vi "Get ASCII string.vi"(8 "error in (no error)":errorcluster, 11 "VISA resource name":refnum<visa-resource-name>) -> (0 "error out":errorcluster, 2 "String":string, 3 "VISA resource name out":refnum<visa-resource-name>)   [LabVIEW 2012, in "Datron D4xxx.lvlib"]
doc: "This VI returns stored ASCII string (X8 command)."
uses:
  Datron D4xxx.lvlib
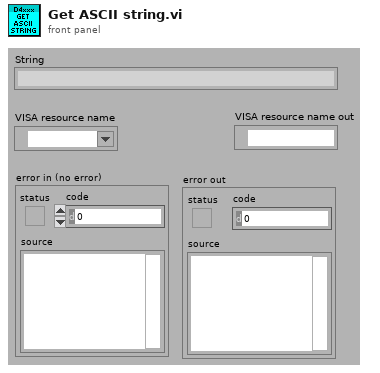
[diagram p1: front panel]
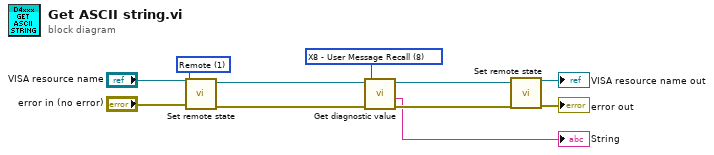
[diagram p0: block diagram]
diagram:
  w6 = u16 8 items=["X0 - Zero Cal Store", "X1 - Gain Cal Store", "X2 - STD Cal Gain Factor", "X3 - Zero Offset", "X4 - Gain Offset", "X5 - Linearity", "X6 - Reference Divider Setting", "X7 - Spot Freq. Corrections", "X8 - User Message Recall", "X9 - Recall Cal Store Selection"] ("X command (X8)")
  w7 = u16 1 items=["Local", "Remote", "Default"] ("Remote state")
  n1 = call "Set remote state.vi"("error in"="error in (no error)", "Remote state"=w7, "VISA resource name"="VISA resource name") -> ("error out"=w4:errorcluster, "VISA resource name out"=w5:refnum<visa-resource-name>)  [unwired: 7 in]
  n2 = call "Get diagnostic value.vi"("error in (no error)"=w4, "X command (X8)"=w6, "VISA resource name"=w5) -> ("error out"=w3:errorcluster, "Respond string"=→"String":string, "VISA resource name out"=w2:refnum<visa-resource-name>)  [unwired: 5 in, 1 out]
  n3 = call "Set remote state.vi"("error in"=w3, "VISA resource name"=w2) -> ("error out"=→"error out":errorcluster, "VISA resource name out"=→"VISA resource name out":refnum<visa-resource-name>)  [unwired: 8 in]
